vi "Settings.vi"(8 "error in (no error)":errorcluster, 9 "Gantry Region":i32=3, 11 "Workspace in":refnum<class "Current Position.lvclass">) -> (0 "error out":errorcluster, 3 "Workspace out":refnum<class "Current Position.lvclass">)   [LabVIEW 2020, in "Current Position.lvclass"]
uses:
  Current Position.lvclass
  C:/Users/hep/Documents/CMU gantry/Classes/Workspace/Fixture.lvclass
  Fixture.lvclass/Fixture.ctl
  Write Gantry Region.vi
panel:
  # "Workspace"
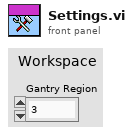
[diagram p1: front panel]
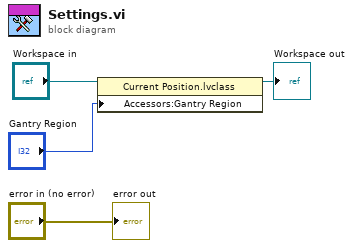
[diagram p0: block diagram]
diagram:
  n1 = property class="Current Position.lvclass"(reference="Workspace in", "Accessors:Gantry Region"="Gantry Region") -> (reference out=→"Workspace out":refnum<class "Current Position.lvclass">)  [unwired: 1 in, 1 out]
  "error out" <- "error in (no error)"
